vi "Set Hard Reset Status.vi"(8 "error in":errorcluster, 10 "Enable":bool, 11 "TPCANHandle in":T2=81 items=["PCAN_NONEBUS"=0, "PCAN_USBBUS1"=81, "PCAN_USBBUS2"=82, "PCAN_USBBUS3"=83, "PCAN_USBBUS4"=84, "PCAN_USBBUS5"=85, "PCAN_USBBUS6"=86, "PCAN_USBBUS7"=87, "PCAN_USBBUS8"=88, "PCAN_USBBUS9"=1289, "PCAN_USBBUS10"=1290, "PCAN_USBBUS11"=1291, "PCAN_USBBUS12"=1292, "PCAN_USBBUS13"=1293, "PCAN_USBBUS14"=1294, "PCAN_USBBUS15"=1295, "PCAN_USBBUS16"=1296]) -> (0 "error out":errorcluster, 3 "TPCANHandle out":T2=81 items=["PCAN_NONEBUS"=0, "PCAN_USBBUS1"=81, "PCAN_USBBUS2"=82, "PCAN_USBBUS3"=83, "PCAN_USBBUS4"=84, "PCAN_USBBUS5"=85, "PCAN_USBBUS6"=86, "PCAN_USBBUS7"=87, "PCAN_USBBUS8"=88, "PCAN_USBBUS9"=1289, "PCAN_USBBUS10"=1290, "PCAN_USBBUS11"=1291, "PCAN_USBBUS12"=1292, "PCAN_USBBUS13"=1293, "PCAN_USBBUS14"=1294, "PCAN_USBBUS15"=1295, "PCAN_USBBUS16"=1296], 5 "TPCANStatus":T1 items=["PCAN_ERROR_OK"=0, "PCAN_ERROR_XMTFULL"=1, "PCAN_ERROR_OVERRUN"=2, "PCAN_ERROR_BUSLIGHT"=4, "PCAN_ERROR_BUSHEAVY"=8, "PCAN_ERROR_BUSPASSIVE"=262144, "PCAN_ERROR_BUSOFF"=16, "PCAN_ERROR_QRCVEMPTY"=32, "PCAN_ERROR_QOVERRUN"=64, "PCAN_ERROR_QXMTFULL"=128, "PCAN_ERROR_REGTEST"=256, "PCAN_ERROR_NODRIVER"=512, "PCAN_ERROR_HWINUSE"=1024, "PCAN_ERROR_NETINUSE"=2048, "PCAN_ERROR_ILLHW"=5120, "PCAN_ERROR_ILLNET"=6144, "PCAN_ERROR_ILLCLIENT"=7168, "PCAN_ERROR_RESOURCE"=8192, "PCAN_ERROR_ILLPARAMTYPE"=16384, "PCAN_ERROR_ILLPARAMVAL"=32768, "PCAN_ERROR_UNKNOWN"=65536, "PCAN_ERROR_ILLDATA"=131072, "PCAN_ERROR_ILLMODE"=524288, "PCAN_ERROR_CAUTION"=33554432, "PCAN_ERROR_INITIALIZE"=67108864, "PCAN_ERROR_ILLOPERATION"=134217728])   [LabVIEW 2019, in "PCANBasic.lvlib"]
doc: "This parameter allows changing the behavior of the function CAN_Reset. \n\nThis parameter can be used only on initialized channels.\n\nNormally, calling this function causes the receive and send message queues for a PCAN-Channel to be\nemptied. The hardware being represented by the channel is not reset. Activating this\nparameter, allows the function to additionally perform a hardware reset after discarding the\nmessages from the channel’s queues.\n\nNote: Performing a hardware reset causes the CAN transceiver to go bus off for a while. This\ncan disturb the CAN communication for a short time, generating error frames by other\nnodes, and avoiding sending/receiving messages.\n\nThe default value of the hard reset (additional hardware reset) is deactivated\n(PCAN_PARAMETER_OFF). After activating it, the hard resset will be performed by the\nfunction CAN_Reset until it is expressly deactivated, or the channel is disconnected (e.g.,\nusing the function CAN_Uninitialize)."
uses:
  PCANBasic.lvlib
  TPCANHandle.ctl
  TPCANStatus.ctl
  TPCANParameter.ctl
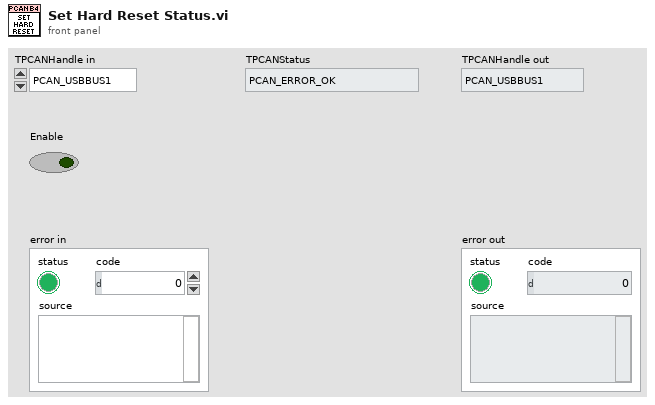
[diagram p1: front panel]
types:
  T1 = typedef "PCANBasic.lvlib/TPCANStatus.ctl" = u32
  T2 = typedef "PCANBasic.lvlib/TPCANHandle.ctl" = u16
  T3 = typedef "PCANBasic.lvlib/TPCANParameter.ctl" = enum16{"Unknown", "PCAN_DEVICE_ID", "PCAN_5VOLTS_POWER", "PCAN_RECEIVE_EVENT", "PCAN_MESSAGE_FILTER", "PCAN_API_VERSION", "PCAN_CHANNEL_VERSION", "PCAN_BUSOFF_AUTORESET", "PCAN_LISTEN_ONLY", "PCAN_LOG_LOCATION", "PCAN_LOG_STATUS", "PCAN_LOG_CONFIGURE", "PCAN_LOG_TEXT", "PCAN_CHANNEL_CONDITION", "PCAN_HARDWARE_NAME", "PCAN_RECEIVE_STATUS", "PCAN_CONTROLLER_NUMBER", "PCAN_TRACE_LOCATION", "PCAN_TRACE_STATUS", "PCAN_TRACE_SIZE", "PCAN_TRACE_CONFIGURE", "PCAN_CHANNEL_IDENTIFYING", "PCAN_CHANNEL_FEATURES", "PCAN_BITRATE_ADAPTING", "PCAN_BITRATE_INFO", "PCAN_BITRATE_INFO_FD", "PCAN_BUSSPEED_NOMINAL", "PCAN_BUSSPEED_DATA", "PCAN_IP_ADDRESS", "PCAN_LAN_SERVICE_STATUS", "PCAN_ALLOW_STATUS_FRAMES", "PCAN_ALLOW_RTR_FRAMES", "PCAN_ALLOW_ERROR_FRAMES", "PCAN_INTERFRAME_DELAY", "PCAN_ACCEPTANCE_FILTER_11BIT", "PCAN_ACCEPTANCE_FILTER_29BIT", "PCAN_IO_DIGITAL_CONFIGURATION", "PCAN_IO_DIGITAL_VALUE", "PCAN_IO_DIGITAL_SET", "PCAN_IO_DIGITAL_CLEAR", "PCAN_IO_ANALOG_VALUE", "PCAN_FIRMWARE_VERSION", "PCAN_ATTACHED_CHANNELS_COUNT", "PCAN_ATTACHED_CHANNELS", "PCAN_ALLOW_ECHO_FRAMES", "PCAN_DEVICE_PART_NUMBER", "PCAN_HARD_RESET_STATUS", "PCAN_LAN_CHANNEL_DIRECTION", "PCAN_DEVICE_GUID"}
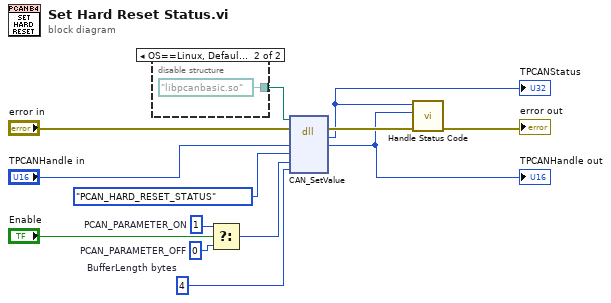
[diagram p0: block diagram]
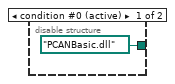
[diagram p2: hidden frame]
diagram:
  w3 = u32 0  # PCAN_PARAMETER_OFF
  w4 = u32 1  # PCAN_PARAMETER_ON
  w8 = u32 4  # BufferLength bytes
  n1 = disable-structure shown="OS==Linux, Default" {
    disable-tunnel: [path "PCANBasic.dll" path "libpcanbasic.so"] -> w13
    frame condition #0 (active) {
    }
    frame condition #1 {
    }
  }
  n2 = Select(t=w4, s="Enable", f=w3) -> (s? t:f=w2:u32)
  n3 = dll-call lib="?" fn="CAN_SetValue"(path in=w13, error in="error in", "Channel"="TPCANHandle in", "TPCANParameter"=TPCANParameter."PCAN_HARD_RESET_STATUS", "Buffer"=w2, "BufferLength"=w8) -> (error out=w10:errorcluster, "TPCANStatus"=w6:u32, "Channel"=w1:u16)  [unwired: 4 in, 1 out]
  "TPCANHandle out" <- w1
  "TPCANStatus" <- w6
  n4 = call "Handle Status Code.vi"("error in"=w10, "TPCANHandle"=w1, "TPCANStatus"=w6) -> ("error out"=→"error out":errorcluster)  [unwired: 8 in]
